vi "Drive Ramp.vi"(8 "MaxDriveIncrement":dbl, 10 "Motor Power":dbl, 11 "Requested  Motor Power in":dbl) -> (3 "Requested  Motor Power out":dbl)   [LabVIEW 2014]
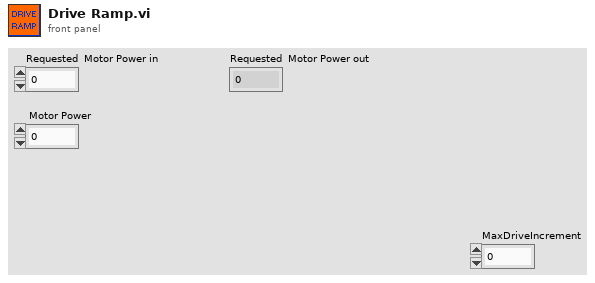
[diagram p1: front panel]
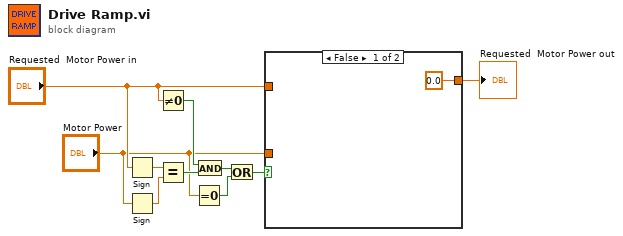
[diagram p0: block diagram]
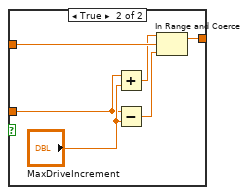
[diagram p2: hidden frame]
diagram:
  n1 = Sign(1:"Requested  Motor Power in") -> (0:w9:dbl)
  n2 = Sign(1:"Motor Power") -> (0:w8:dbl)
  n3 = Not Equal To 0?(x="Requested  Motor Power in") -> (x != 0?=w6:bool)
  n4 = Equal?(x=w9, y=w8) -> (x = y?=w5:bool)
  n5 = Equal To 0?(x="Motor Power") -> (x = 0?=w4:bool)
  n6 = And(x=w6, y=w5) -> (x .and. y?=w2:bool)
  n7 = Or(x=w2, y=w4) -> (x .or. y?=w1:bool)
  n8 = case shown="False" w1 {
    tunnel: "Motor Power" -> [_ w16]
    tunnel: "Requested  Motor Power in" -> [_ w15]
    tunnel: [0.0 ("Requested  Motor Power in") w12] -> w10
    frame False {
    }
    frame True {
      n9 = Add(x=w16, y="MaxDriveIncrement") -> (x+y=w14:dbl)
      n10 = Subtract(x=w16, y="MaxDriveIncrement") -> (x-y=w13:dbl)
      n11 = In Range and Coerce(upper limit=w14, x=w15, lower limit=w13) -> (coerced(x)=w12:dbl)  [unwired: 1 out]
    }
  }
  "Requested  Motor Power out" <- w10
